vi "TCP Read Bytes.vi"(8 "error in (no error)":errorcluster, 9 "timeout (1000 ms)":i32=1000, 10 "bytes to read (100)":i32=100, 11 "Connection.TCP":refnum<class "Connection.TCP.lvclass">) -> (0 "error out":errorcluster, 1 "timed out":bool, 2 "Bytes":u8[](array[numeric]) format="%08b", 3 "Connection.TCP":refnum<class "Connection.TCP.lvclass">, 4 "connected":bool)   [LabVIEW 2013, in "Connection.TCP_GOSPL.lvlib" / "Connection.TCP.lvclass"]
uses:
  Connection.TCP.lvclass
  Connection.TCP.lvclass/Connection.TCP.ctl
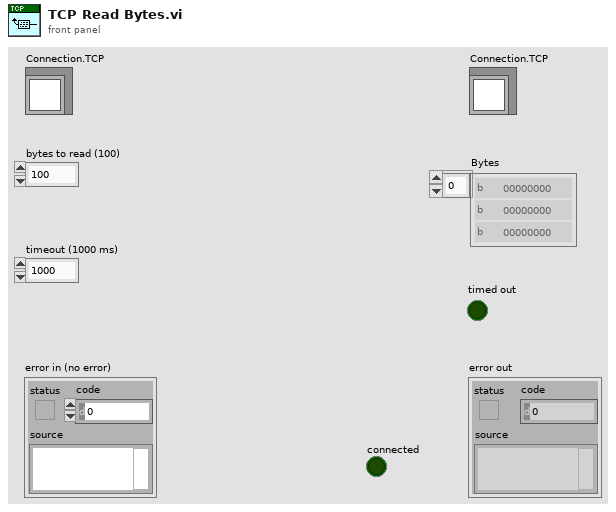
[diagram p1: front panel]
types:
  T1 = enum16{"Standard", "Buffered", "CRLF", "Immediate"}
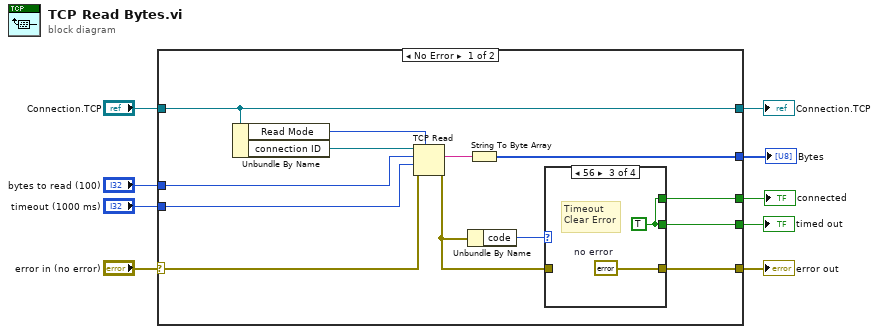
[diagram p0: block diagram]
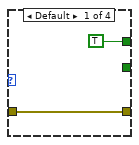
[diagram p2: hidden frame]
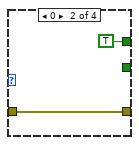
[diagram p3: hidden frame]
diagram:
  n1 = case shown="No Error" "error in (no error)" {
    selector: "error in (no error)" -> [w21 w31]
    tunnel: [w12 w31] -> w8
    tunnel: [w13 w30] -> w6
    tunnel: "Connection.TCP" -> [w13 w30]
    tunnel: [w19 _] -> w5
    tunnel: "bytes to read (100)" -> [w16 _]
    tunnel: "timeout (1000 ms)" -> [w15 _]
    tunnel: [w14 _] -> w2
    tunnel: [w11 _] -> w1
    frame No Error {
      n2 = Unbundle By Name(w13) -> ("Read Mode"=w10:T1, "connection ID"=w22:refnum<k5>)
      n3 = TCP Read(connection ID=w22, bytes to read=w16, error in (no error)=w21, 7:w10, 9:w15) -> (data out=w20:string, error out=w17:errorcluster)  [unwired: 1 out]
      n4 = Unbundle By Name(w17) -> ("code"=w18:i32)
      n5 = String To Byte Array(string=w20) -> (unsigned byte array=w19:u8[])
      n6 = case shown="56" w18 {
        tunnel: [w24 w26 w27 w29] -> w12
        tunnel: w17 -> [w24 w26 _ w29]
        tunnel: [_ _ w28 _] -> w14
        tunnel: [TRUE TRUE w28 _] -> w11
        frame Default {
        }
        frame 0 {
        }
        frame 56 {
          w27 = errorcluster {"status"=FALSE, "code"=0, "source"=""}  # no error
          w28 = TRUE
          # "Timeout\nClear Error"
        }
        frame 66 {
          # "Disconnection\nby peer"
        }
      }
    }
    frame Error {
    }
  }
  "error out" <- w8
  "Connection.TCP" <- w6
  "Bytes" <- w5
  "timed out" <- w2
  "connected" <- w1
